vi "Set Control Mode.vi"(8 "error in (no error)":errorcluster, 10 "Internal Control":bool, 11 "VISA session":refnum<visa-resource-name>) -> (0 "error out":errorcluster, 3 "dup VISA session":refnum<visa-resource-name>)   [LabVIEW 2018, in "Lauda TCU.lvlib"]
uses:
  Lauda TCU.lvlib
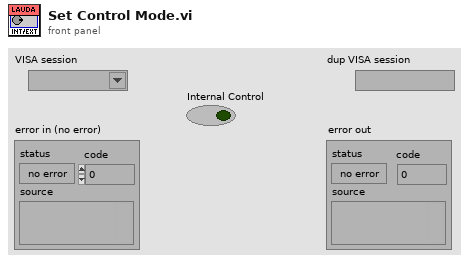
[diagram p1: front panel]
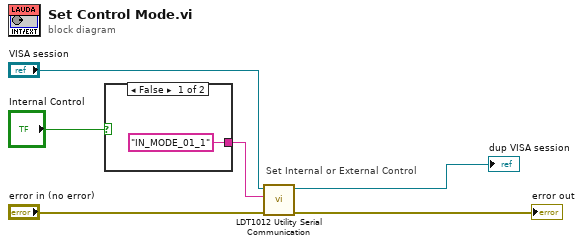
[diagram p0: block diagram]
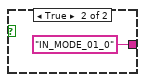
[diagram p2: hidden frame]
diagram:
  # "Set Internal or External Control"
  n1 = case shown="False" "Internal Control" {
    tunnel: ["IN_MODE_01_1" "IN_MODE_01_0"] -> w6
    frame False {
    }
    frame True {
    }
  }
  n2 = call "LDT1012 Utility Serial Communication.vi"("error in (no error)"="error in (no error)", "Command String"=w6, "VISA session"="VISA session") -> ("error out"=→"error out":errorcluster, "dup VISA session"=→"dup VISA session":refnum<visa-resource-name>)  [unwired: 5 in, 2 out]
